vi "Stop Core.vi"(6 "final error code":i32, 11 "Mediated Asynchronous Actor in":refnum<class "Mediated Asynchronous Actor.lvclass">) -> (3 "Mediated Asynchronous Actor out":refnum<class "Mediated Asynchronous Actor.lvclass">)   [LabVIEW 2016, in "Stream Mediator.lvlib" / "Mediated Asynchronous Actor.lvclass"]
doc: "--\nCopyright © 2017 Composed SystemsI All rights reserved.\n\nAuthor: Jon McBee <jon.mcbee@composed.io>\n\nThis library is provided \"AS IS\" ,WITHOUT WARRANTIES OR\nCONDITIONS OF ANY KIND, either express or implied.\n\nComposed Systems -- composed.io\n\nStream 0.0.1.1\nJon McBee - Composed Systems\nCopyright (c) 2017, Composed Systems"
uses:
  <userlib>/Composed Systems/Stream/Mediator/Classes/Mediated Asynchronous Actor/Mediated Asynchronous Actor.lvclass
  C:/Program Files (x86)/National Instruments/LabVIEW 2016/user.lib/Composed Systems/Stream/Actor/Actor Class/Ancestral Actor.lvclass
  <userlib>/Composed Systems/Stream/Mediator/Classes/Message Transport Interface/Message Priority.ctl
  <userlib>/Composed Systems/Stream/Actor/Actor Class/Ancestral Actor.lvclass/Ancestral Actor.ctl
  <userlib>/Composed Systems/Stream/Mediator/Classes/Mediated Asynchronous Actor/Mediated Asynchronous Actor.lvclass/Mediated Asynchronous Actor.ctl
  <userlib>/Composed Systems/Stream/Mediator/Classes/Message Transport Interface/Message Transport Interface.lvclass
  <userlib>/Composed Systems/Stream/Mediator/Classes/Message Command Stop/Stop Msg.lvclass
  <userlib>/Composed Systems/Stream/Actor/Actor Class/Ancestral Actor.lvclass
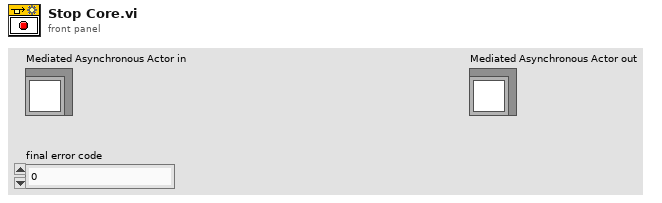
[diagram p1: front panel]
types:
  T1 = typedef "Stream Mediator.lvlib/Message Transport Interface.lvclass/Message Priority.ctl" = enum16{"Normal", "High"}
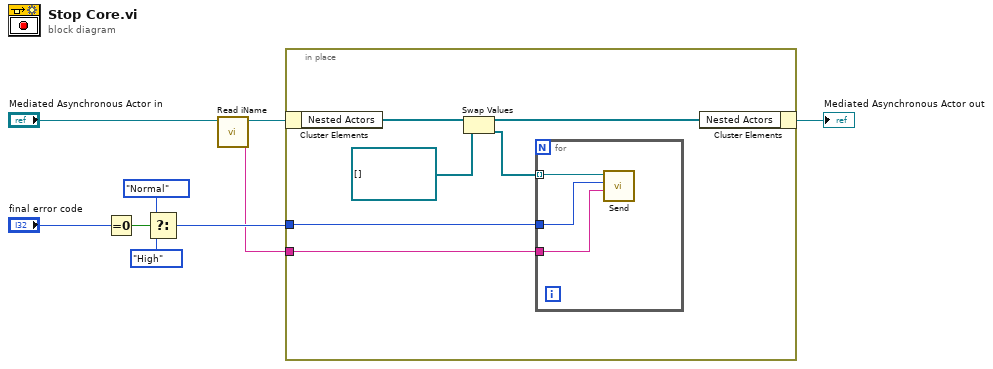
[diagram p0: block diagram]
diagram:
  n1 = Equal To 0?(x="final error code") -> (x = 0?=w9:bool)
  n2 = Select(t=Message_Priority."Normal", s=w9, f=Message_Priority."High" ("Message Priority")) -> (s? t:f=w5:T1)
  n3 = call <userlib>:"Read iName.vi"("Ancestral Actor in"="Mediated Asynchronous Actor in") -> ("iName"=w1:string, "Ancestral Actor out"=w2:refnum<class "Mediated Asynchronous Actor.lvclass">)  [unwired: 8 in, 1 out]
  n4 = in-place {
    in-place-border: w5 -> [w11]
    in-place-border: w1 -> [w10]
    n5 = in-place-cluster #1(w2) -> ("Nested Actors"=w15:refnum<class "Message Transport Interface.lvclass">[])
    n6 = Swap Values(12:w15, 14:refnum<class "Message Transport Interface.lvclass">[] [] ("Nested Actors")) -> (1:w13:refnum<class "Message Transport Interface.lvclass">[], 3:w12:refnum<class "Message Transport Interface.lvclass">[])  [unwired: 1 in]
    n7 = for {
      tunnel: w12 -> [w18] mode=indexing
      tunnel: w11 -> [w17]
      tunnel: w10 -> [w16]
      n8 = call <userlib>:"Send.vi"("Caller Actor Name"=w16, "Message Priority"=w17, "Message Transport"=w18) -> ()  [unwired: 8 in, 1 out]
    }
    n9 = in-place-cluster #1("Nested Actors"=w13) -> (→"Mediated Asynchronous Actor out":refnum<class "Mediated Asynchronous Actor.lvclass">)
  }
